vi "New.vi"() -> (0 "Null":refnum<class "Null.lvclass">)   [LabVIEW 2018, in "Toolkit.lvlib" / "Data.lvlib" / "Null.lvclass"]
doc: "Creates a new Mustache NULL data type object. Generally, if the Mustache data is NULL, then Mustache template tag will not be rendered."
uses:
  Null.lvclass
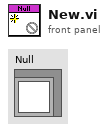
[diagram p1: front panel]
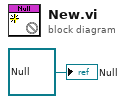
[diagram p0: block diagram]
diagram:
  "Null" <- refnum<class "Null.lvclass"> refnum ("Toolkit.lvlib:Types.lvlib:Null.lvclass")
